vi "Untitled 5.vi"() -> ()   [LabVIEW 2015]
panel:
  out "timed out?\nBattery Potentiometer\nPotentiometer":bool
  out "Battery Potentiometer\nPotentiometer (3202)":sgl
  out "Low Battery\nfor Potentiometer sensor":errorcluster
  # "Battery potentiometer"
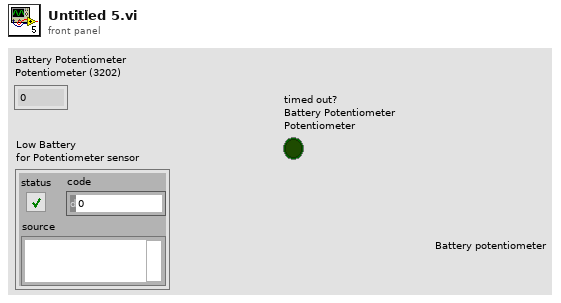
[diagram p1: front panel]
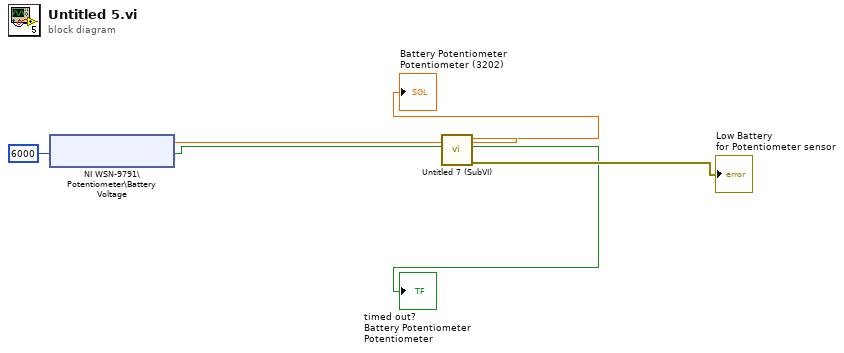
[diagram p0: block diagram]
diagram:
  n1 = shared-variable "NI WSN-9791\\Potentiometer\\Battery Voltage"(6000 ("ms timeout (0)")) -> (w4:sgl, w5:bool)  [unwired: 1 in, 1 out]
  n2 = call "Untitled 7 (SubVI).vi"("Boolean"=w5, "Numeric"=w4) -> ("error out"=→"Low Battery\nfor Potentiometer sensor":errorcluster, "timed out?\nBattery Potentiometer\nPotentiometer"=→"timed out?\nBattery Potentiometer\nPotentiometer":bool, "Battery Potentiometer\nPotentiometer (3202)"=→"Battery Potentiometer\nPotentiometer (3202)":sgl)  [unwired: 7 in]
